vi "VMC_setup.vi"(0 "PnaVisa":refnum<visa-resource-name>="PNA", 5 "Mixer file (*.mxr)":path, 7 "Format":string(combo)="MLINear", 9 "Measurement":string(combo)="VC21", 11 "error in":errorcluster, 12 "Channel":i32=1) -> (4 "dup VISA session":refnum<visa-resource-name>, 8 "FileName":string="Mixer", 15 "error out":errorcluster)   [LabVIEW 2018]
uses:
  Instance           2 17Saved   VMC_setup .vi
  Instance           1 17Saved   VMC_setup .vi
  PNA-X.lvlib
panel:
  # "The Mixer file must be stored locally on the PNA"
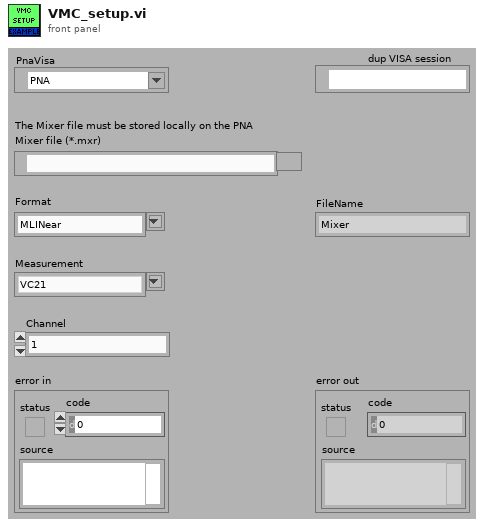
[diagram p1: front panel]
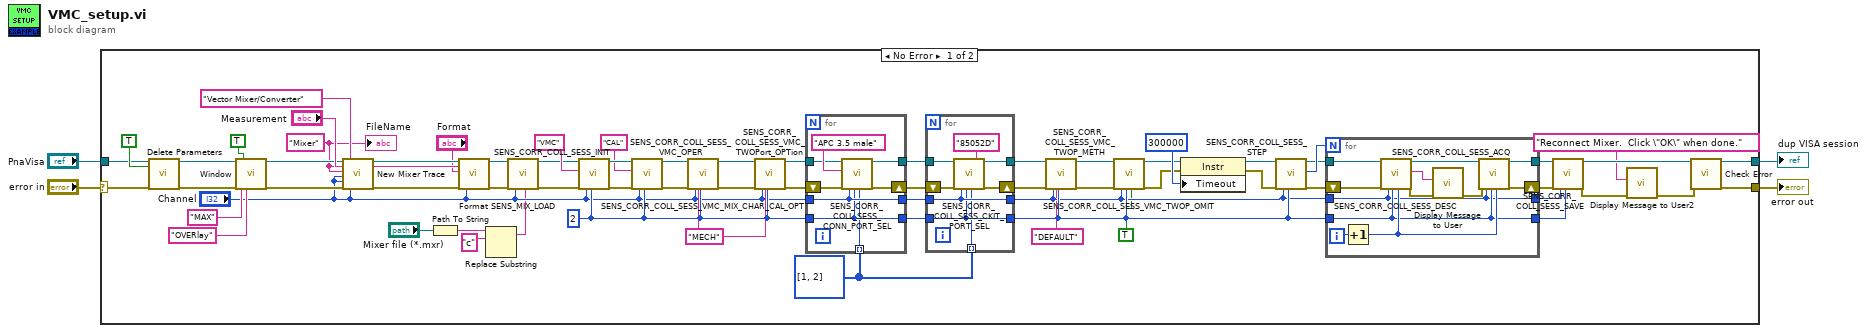
[diagram p0: block diagram]
diagram:
  n1 = case shown="No Error" "error in" {
    selector: "error in" -> [w9 w102]
    tunnel: "PnaVisa" -> [w71 w101]
    tunnel: [w58 w102] -> w3
    tunnel: [w57 w101] -> w2
    frame No Error {
      w32 = i32[] [1, 2]
      w22 = 2
      w21 = "MECH" ("CalType")
      w15 = "Mixer" ("FileName")
      n2 = call "Delete Parameters .vi"("VISA IN"=w71, "Delete All?"=TRUE, "error in"=w9) -> ("VISA Out"=w70:refnum<visa-resource-name>, "error out"=w69:errorcluster)  [unwired: 15 in]
      n3 = call "Window.vi"("VISA IN"=w70, "error in"=w69, "Window\nCreate(ON)/Delete(OFF)"=TRUE ("Window\nCreate(ON)/Delete(OFF)"), "Window Size"="MAX", "Window Arrangement"="OVERlay") -> ("VISA Out"=w51:refnum<visa-resource-name>, "error out"=w52:errorcluster)  [unwired: 13 in]
      n4 = call "New Mixer Trace.vi"("VISA IN"=w51, "Meas Param"="Measurement", "FileName"=w15, "Window"="Channel", "Trace"="Channel", "error in (no error)"=w52, "Meas Type"="Vector Mixer/Converter" ("Measurement Type"), "Channel"="Channel") -> ("VISA Out"=w20:refnum<visa-resource-name>, "error out"=w19:errorcluster)  [unwired: 10 in]
      n5 = Path To String(path="Mixer file (*.mxr)") -> (string=w13:string)
      n6 = call "Format.vi"("VISA IN"=w20, "Measurement Name"=w15, "Format"="Format", "error in"=w19, "Channel"="Channel") -> ("VISA Out"=w18:refnum<visa-resource-name>, "error out"=w17:errorcluster)  [unwired: 13 in]
      n7 = Replace Substring(4:"c" ("substring (\"\")"), 5:w13) -> (1:w10:string)  [unwired: 2 in, 1 out]
      n8 = call "SENS_MIX_LOAD.vi"("VISA IN"=w18, "error in"=w17, "Channel"="Channel", "FileName"=w10) -> ("VISA Out"=w50:refnum<visa-resource-name>, "error out"=w49:errorcluster)  [unwired: 14 in]
      n9 = call "SENS_CORR_COLL_SESS_INIT.vi"("VISA IN"=w50, "ClaType"="VMC", "error in"=w49, "Channel"="Channel", "Session"=w22) -> ("VISA Out"=w37:refnum<visa-resource-name>, "error out"=w40:errorcluster)  [unwired: 13 in]
      n10 = call "SENS_CORR_COLL_SESS_VMC_OPER.vi"("VISA IN"=w37, "CalType"="CAL", "error in"=w40, "Channel"="Channel", "Session"=w22) -> ("VISA Out"=w38:refnum<visa-resource-name>, "error out"=w39:errorcluster)  [unwired: 13 in]
      n11 = call "SENS_CORR_COLL_SESS_VMC_MIX_CHAR_CAL_OPT.vi"("VISA IN"=w38, "error in"=w39, "Channel"="Channel", "Session"=w22, "CalType"=w21) -> ("VISA Out"=w41:refnum<visa-resource-name>, "error out"=w42:errorcluster)  [unwired: 13 in]
      n12 = call "SENS_CORR_COLL_SESS_VMC_TWOPort_OPTion.vi"("VISA IN"=w41, "error in"=w42, "Channel"="Channel", "Session"=w22, "CalType"=w21) -> ("VISA Out"=w47:refnum<visa-resource-name>, "error out"=w48:errorcluster)  [unwired: 13 in]
      n13 = for {
        tunnel: [w80] -> w31
        shift-right: [w78] -> w30
        shift-left: w48 -> [w79]
        tunnel: "Channel" -> [w77]
        tunnel: [w77] -> w34
        tunnel: w22 -> [w76]
        tunnel: [w76] -> w33
        tunnel: w32 -> [w74] mode=indexing
        tunnel: w47 -> [w73]
        n14 = call "SENS_CORR_COLL_SESS_CONN_PORT_SEL.vi"("VISA IN"=w73, "ConnType"="APC 3.5 male", "error in"=w79, "Channel"=w77, "Session"=w76, "Port"=w74) -> ("VISA Out"=w80:refnum<visa-resource-name>, "error out"=w78:errorcluster)  [unwired: 12 in]
      }
      n15 = for {
        shift-right: [w85] -> w29
        shift-left: w30 -> [w88]
        tunnel: w34 -> [w84]
        tunnel: w33 -> [w83]
        tunnel: w32 -> [w81] mode=indexing
        tunnel: [w87] -> w28
        tunnel: [w84] -> w54
        tunnel: [w83] -> w55
        tunnel: w31 -> [w82]
        n16 = call "SENS_CORR_COLL_SESS_CKIT_PORT_SEL.vi"("VISA IN"=w82, "error in"=w88, "Channel"=w84, "Session"=w83, "Port"=w81, "CalKit"="85052D") -> ("VISA Out"=w87:refnum<visa-resource-name>, "error out"=w85:errorcluster)  [unwired: 12 in]
      }
      n17 = call "SENS_CORR_COLL_SESS_VMC_TWOP_METH.vi"("VISA IN"=w28, "error in"=w29, "Channel"=w54, "Session"=w55, "Method"="DEFAULT") -> ("VISA Out"=w25:refnum<visa-resource-name>, "error out"=w26:errorcluster)  [unwired: 13 in]
      n18 = call "SENS_CORR_COLL_SESS_VMC_TWOP_OMIT.vi"("VISA IN"=w25, "error in"=w26, "Channel"=w54, "Session"=w55, "OmitIsol?"=TRUE) -> ("VISA Out"=w46:refnum<visa-resource-name>, "error out"=w45:errorcluster)  [unwired: 13 in]
      n19 = property class="Instr"(reference=w46, error in=w45, "Timeout"=u32 300000 ("General Settings:Timeout Value")) -> (reference out=w43:refnum<visa-resource-name>, error out=w44:errorcluster)
      n20 = call "SENS_CORR_COLL_SESS_STEP.vi"("VISA IN"=w43, "error in"=w44, "Channel"=w54, "Session"=w55) -> ("VISA Out"=w23:refnum<visa-resource-name>, "Step"=w63:i32, "error out"=w24:errorcluster)  [unwired: 13 in]
      n21 = for {
        N: w63 -> [_]
        tunnel: w23 -> [w99]
        shift-right: [w94] -> w61
        shift-left: w24 -> [w98]
        tunnel: [w95] -> w62
        tunnel: w55 -> [w92]
        tunnel: [w92] -> w60
        tunnel: w54 -> [w91]
        tunnel: [w91] -> w53
        i -> [w100]
        n22 = Increment(x=w100) -> (x+1=w93:i32)
        n23 = call "SENS_CORR_COLL_SESS_DESC.vi"("VISA IN"=w99, "error in"=w98, "Channel"=w91, "Session"=w92, "StepNum"=w93) -> ("VISA Out"=w96:refnum<visa-resource-name>, "read buffer"=w97:string, "error out"=w90:errorcluster)  [unwired: 12 in]
        n24 = call "Display Message to User"("error in (no error)"=w90, "Message"=w97) -> ("error out"=w89:errorcluster)  [unwired: 8 in, 1 out]
        n25 = call "SENS_CORR_COLL_SESS_ACQ.vi"("VISA IN"=w96, "error in"=w89, "Channel"=w91, "Session"=w92, "AcqCnt"=w93) -> ("VISA Out"=w95:refnum<visa-resource-name>, "error out"=w94:errorcluster)  [unwired: 13 in]
      }
      n26 = call "SENS_CORR_COLL_SESS_SAVE.vi"("VISA IN"=w62, "error in"=w61, "Channel"=w53, "Session"=w60) -> ("VISA Out"=w6:refnum<visa-resource-name>, "error out"=w8:errorcluster)  [unwired: 14 in]
      n27 = call "Display Message to User2"("error in (no error)"=w8, "Message"="Reconnect Mixer.  Click \"OK\" when done.") -> ("error out"=w7:errorcluster)  [unwired: 8 in, 1 out]
      n28 = call "Check Error.vi"("VISA Resource Name"=w6, "error in (no error)"=w7) -> ("dup VISA session"=w57:refnum<visa-resource-name>, "error out"=w58:errorcluster)  [unwired: 16 in]
      "FileName" <- w15
    }
    frame Error {
    }
  }
  "error out" <- w3
  "dup VISA session" <- w2
